vi "Twitter Open - Desktop.vi"(8 "error in":errorcluster, 9 "Access Credentials (in)":T1, 10 "Consumer Secret":string, 11 "Consumer Key":string) -> (0 "error out":errorcluster, 1 "Access Credentials (out)":T1, 3 "Twitter Handle Out":T2={"OAuth Credentials"={"Signature Method"=enum."HMAC-SHA1", "Version"="1.0", "Client"={"Token"="", "Secret"=""}, "Access"={"Token"="", "Secret"=""}}, "since ID"="", "max ID"="", "Screen Name"=""})   [LabVIEW 2011, in "i3-twitter.lvlib"]
doc: "<b>Twitter Open - Desktop</b> is used on Desktops with a Web Browser installed to connect to Twitter and verify that the user credentials are valid. If the user approves the application or the provided Access Credentials are valid then a Twitter Handle is returned. Applications run on platforms without Desktops or that require a specific fixed set of Access Tokens should use <b>Twitter Open - Embedded</b>.\n\nThe <b>Consumer Key</b> and <b>Consumer Secret</b> are unique to each application and can be created by making an application at dev.twitter.com. For more information and a Getting Started tutorial navigate to Help » i3 Twitter Help in LabVIEW.\n\n<b>Access Credentials</b> are created when the user runs Twitter Open and the user approves the application request. Save the Access Credentials and in the future when Twitter Open is called the Access Credentials can be provided to prevent the user from having to log in repeatedly."
uses:
  i3-twitter.lvlib
  Controls/Twitter Handle.ctl
  i3-oauth/Controls/OAuth Handle.ctl
  i3-oauth/Controls/Signature Method.ctl
  i3-oauth/Controls/Credentials.ctl
  <vilib>/Utility/error.llb/whitespace.ctl
  i3-oauth/Controls/Authorization URLs.ctl
  i3-oauth/i3-oauth.lvlib
panel:
  out "Response Header":string
  out "Response Body":string
  # "Debug Only"
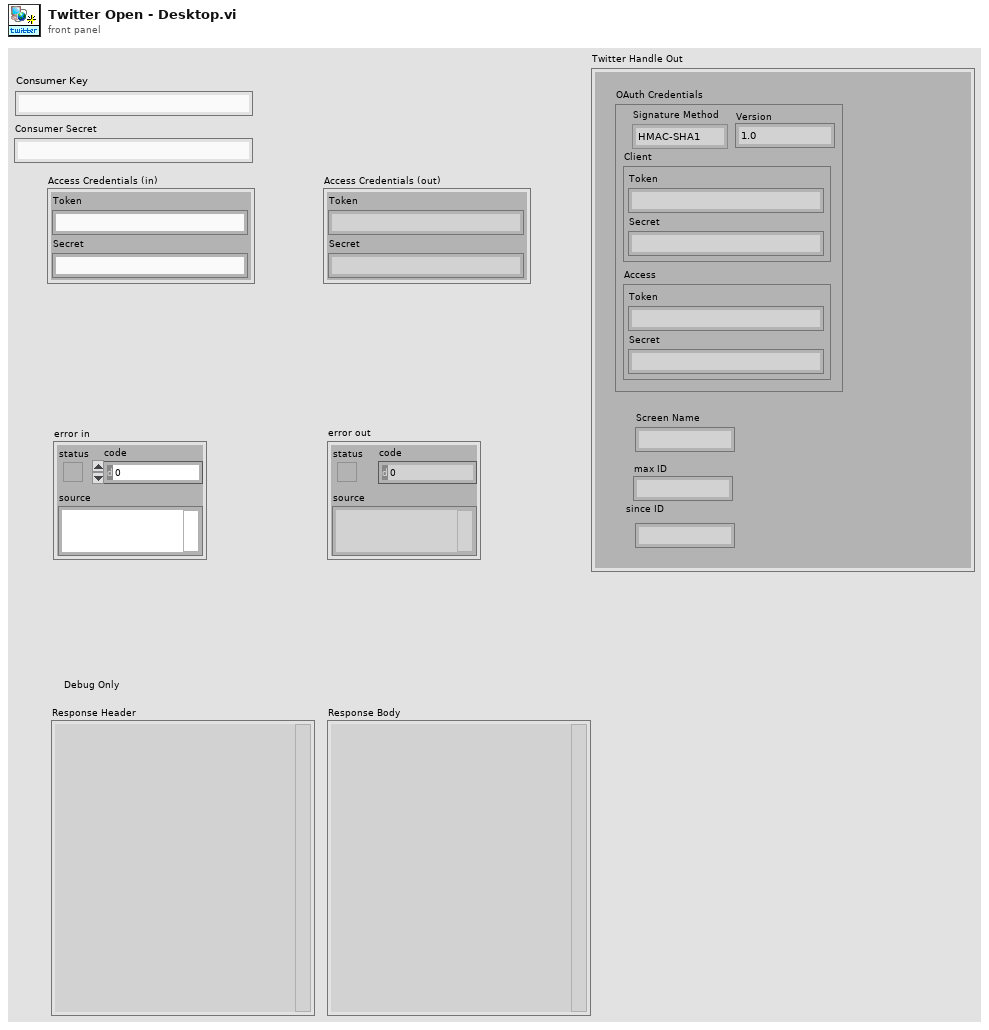
[diagram p1: front panel]
types:
  T1 = typedef "i3-oauth.lvlib/Credentials.ctl" = cluster{"Token":string, "Secret":string}
  T2 = typedef "i3-twitter.lvlib/Twitter Handle.ctl" = cluster{"OAuth Credentials":T3, "since ID":string, "max ID":string, "Screen Name":string}
  T3 = typedef "i3-oauth.lvlib/OAuth Handle.ctl" = cluster{"Signature Method":T4, "Version":string, "Client":T1, "Access":T1}
  T4 = typedef "i3-oauth.lvlib/Signature Method.ctl" = enum16{"HMAC-MD5", "HMAC-SHA1", "HMAC-SHA224", "HMAC-SHA256", "HMAC-SHA384", "HMAC-SHA512"}
  T5 = typedef "i3-oauth.lvlib/Authorization URLs.ctl" = cluster{"Request URL":string, "Authorize URL":string, "Access URL":string}
  T6 = typedef "whitespace.ctl" = u16
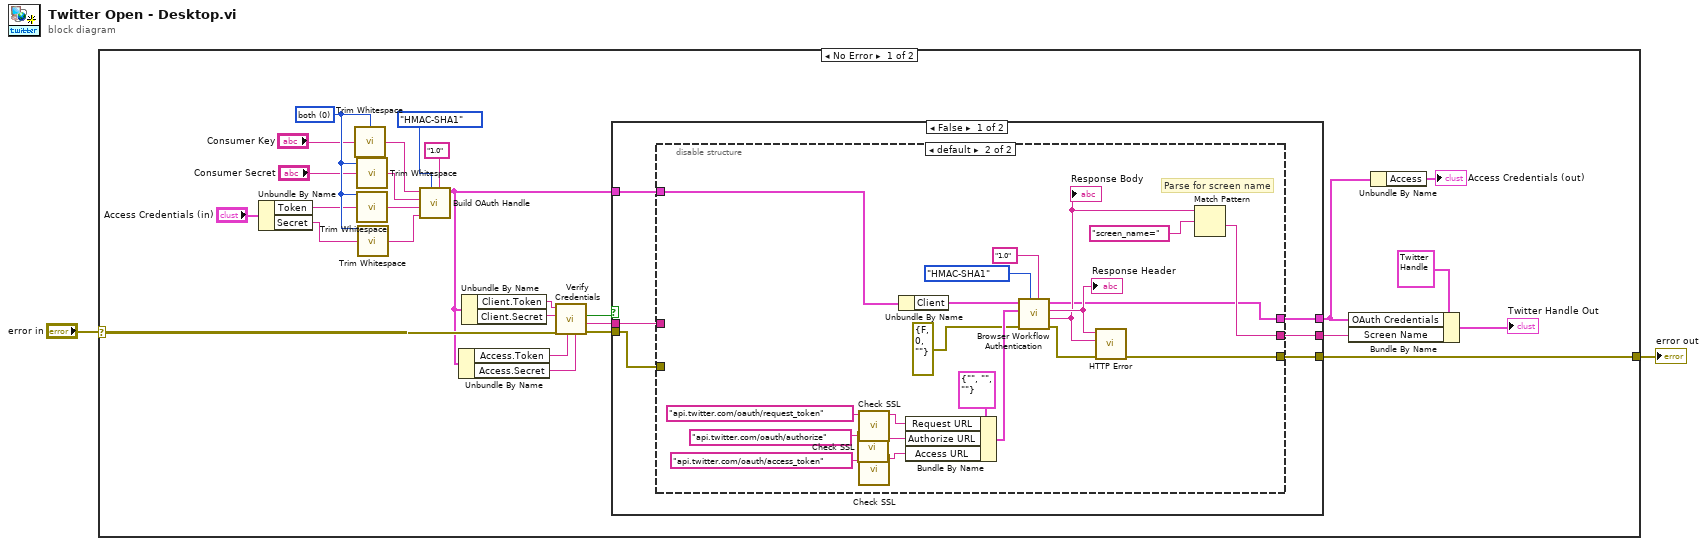
[diagram p0: block diagram]
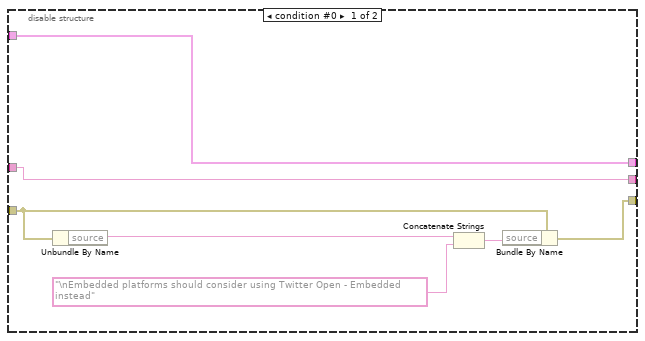
[diagram p2: hidden frame]
diagram:
  n1 = case shown="No Error" "error in" {
    selector: "error in" -> [w20 w66]
    tunnel: [w27 w66] -> w2
    frame No Error {
      w29 = T6 0 items=["both", "start of string", "end of string"] ("location (both)")
      n2 = Unbundle By Name("Access Credentials (in)") -> ("Token"=w7:string, "Secret"=w9:string)
      n3 = call <vilib>:"Trim Whitespace.vi"("string"="Consumer Key", "location (both)"=w29) -> ("trimmed string"=w4:string)
      n4 = call <vilib>:"Trim Whitespace.vi"("string"="Consumer Secret", "location (both)"=w29) -> ("trimmed string"=w6:string)
      n5 = call <vilib>:"Trim Whitespace.vi"("string"=w7, "location (both)"=w29) -> ("trimmed string"=w8:string)
      n6 = call <vilib>:"Trim Whitespace.vi"("string"=w9, "location (both)"=w29) -> ("trimmed string"=w10:string)
      n7 = call "Build OAuth Handle.vi"("Version (1.0)"="1.0", "Signature Method (HMAC-SHA1)"=Signature_Method."HMAC-SHA1", "Access Secret"=w10, "Access Token"=w8, "Client Secret"=w6, "Client Token"=w4) -> ("OAuth Handle"=w11:T3)  [unwired: 5 in]
      n8 = Unbundle By Name(w11) -> ("Access.Token"=w13:string, "Access.Secret"=w12:string)
      n9 = Unbundle By Name(w11) -> ("Client.Token"=w14:string, "Client.Secret"=w15:string)
      n10 = call "Verify Credentials.vi"("Access Token Secret (In)"=w12, "Access Token (In)"=w13, "error in (no error)"=w20, "Consumer Secret"=w15, "Consumer Key"=w14) -> ("error out"=w24:errorcluster, "Screen Name"=w23:string, "Success?"=w28:bool)  [unwired: 3 in, 1 out]
      n11 = case shown="False" w28 {
        tunnel: [w33 w63] -> w22
        tunnel: [w34 w65] -> w27
        tunnel: [w35 w64] -> w25
        tunnel: w24 -> [w30 w65]
        tunnel: w23 -> [w31 w64]
        tunnel: w11 -> [w32 w63]
        frame False {
          n12 = disable-structure shown="default" {
            disable-tunnel: [w41 w62] -> w35
            disable-tunnel: [w40 w60] -> w34
            disable-tunnel: [w42 w53] -> w33
            disable-tunnel: w32 -> [w42 w47]
            disable-tunnel: w31 -> [w41 _]
            disable-tunnel: w30 -> [w39 _]
            frame condition #0 {
              n13 = Unbundle By Name(w39) -> ("source"=w37:string)
              n14 = Concatenate Strings(w37, "\nEmbedded platforms should consider using Twitter Open - Embedded instead" ("string")) -> (w38:string)
              n15 = Bundle By Name(cluster=w39, "source"=w38) -> (w40:errorcluster)
            }
            frame condition #1 (active) {
              # "Parse for screen name"
              n16 = call "Check SSL.vi"("Input URL"="api.twitter.com/oauth/authorize" ("Authorize URL")) -> ("Output URL"=w50:string)  [unwired: 8 in]
              n17 = call "Check SSL.vi"("Input URL"="api.twitter.com/oauth/request_token" ("Request URL")) -> ("Output URL"=w51:string)  [unwired: 8 in]
              n18 = call "Check SSL.vi"("Input URL"="api.twitter.com/oauth/access_token" ("Access URL")) -> ("Output URL"=w49:string)  [unwired: 8 in]
              n19 = Unbundle By Name(w47) -> ("Client"=w46:T1)
              n20 = Bundle By Name(cluster=T5 {"Request URL"="", "Authorize URL"="", "Access URL"=""} ("Authorization URLs"), "Request URL"=w51, "Authorize URL"=w50, "Access URL"=w49) -> (w48:T5)
              n21 = call "Browser Workflow Authentication.vi"("Version (1.0)"="1.0", "Signature Method (HMAC-SHA1)"=Signature_Method."HMAC-SHA1", "error in (no error)"=errorcluster {"status"=FALSE, "code"=0, "source"=""}, "Authorization URLs"=w48, "Client Credentials"=w46) -> ("error out"=w61:errorcluster, "Access Response Body"=w54:string, "Access Response Header"=w55:string, "OAuth Handle"=w53:T3)  [unwired: 3 in]
              "Response Body" <- w54
              "Response Header" <- w55
              n22 = call "HTTP Error.vi"("error in (no error)"=w61, "Body"=w54, "Header"=w55) -> ("error out"=w60:errorcluster)  [unwired: 6 in, 2 out]
              n23 = Match Pattern(string=w54, regular expression="screen_name=" ("format string")) -> (after substring=w62:string)  [unwired: 1 in, 3 out]
            }
          }
        }
        frame True {
        }
      }
      n24 = Bundle By Name(cluster=T2 {"OAuth Credentials"={"Signature Method"=enum."HMAC-MD5", "Version"="", "Client"={"Token"="", "Secret"=""}, "Access"={"Token"="", "Secret"=""}}, "since ID"="", "max ID"="", "Screen Name"=""} ("Twitter Handle"), "OAuth Credentials"=w22, "Screen Name"=w25) -> (→"Twitter Handle Out":T2)
      n25 = Unbundle By Name(w22) -> ("Access"=→"Access Credentials (out)":T1)
    }
    frame Error {
    }
  }
  "error out" <- w2
